vi "Configure List.vi"(0 "VISA resource name":refnum<visa-resource-name>, 1 "Amplitude Data":dbl[](array[numeric])=[1.0] format="%#.4g", 2 "Trigger Output Data":bool[](array[boolean]), 5 "List Type (0: Current)":u16(ring) items=["Current", "Dwell", "Frequency", "Frequency Slew Rate", "Phase", "Waveform", "Trigger Output", "Voltage", "Voltage Slew Rate", "Voltage Offset", "Voltage Offset Slew Rate"], 7 "List Repeat Count (1)":dbl=1.0, 9 "List Sequencing (0: Auto)":u16(ring) items=["Auto", "Once"], 11 "error in (no error)":errorcluster, 12 "Waveform Data":T1(array[cluster]) {"Shape (0: Sinusoid)" items=["Sinusoid", "Square", "Clipped Sinusoid", "User-Specified"]}) -> (4 "VISA resource name out":refnum<visa-resource-name>, 15 "error out":errorcluster)   [LabVIEW 2019, in "Agilent 681x Series.lvlib"]
doc: "Configures the lists of various parameters such as voltage, current or frequency for the instrument to use when list mode is selected for configuration of those parameters."
uses:
  <instrlib>/Agilent 681x Series/Agilent 681x Series.lvlib
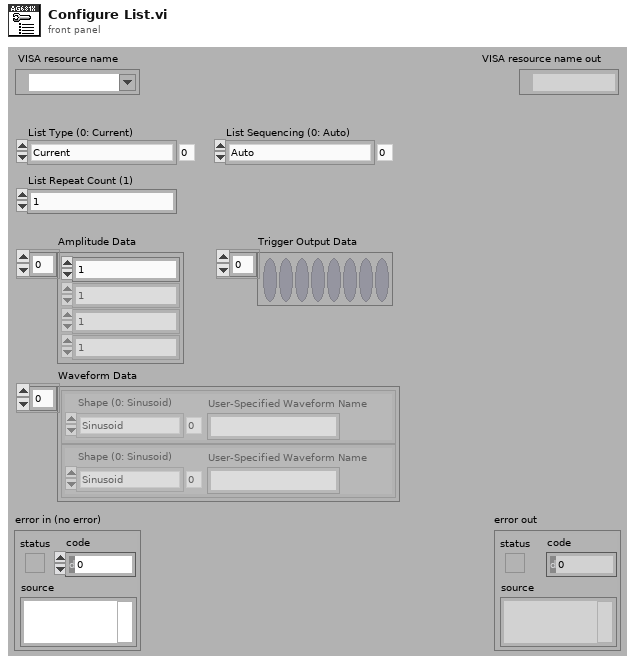
[diagram p1: front panel]
types:
  T1 = cluster{"Shape (0: Sinusoid)":u16, "User-Specified Waveform Name":string}[]
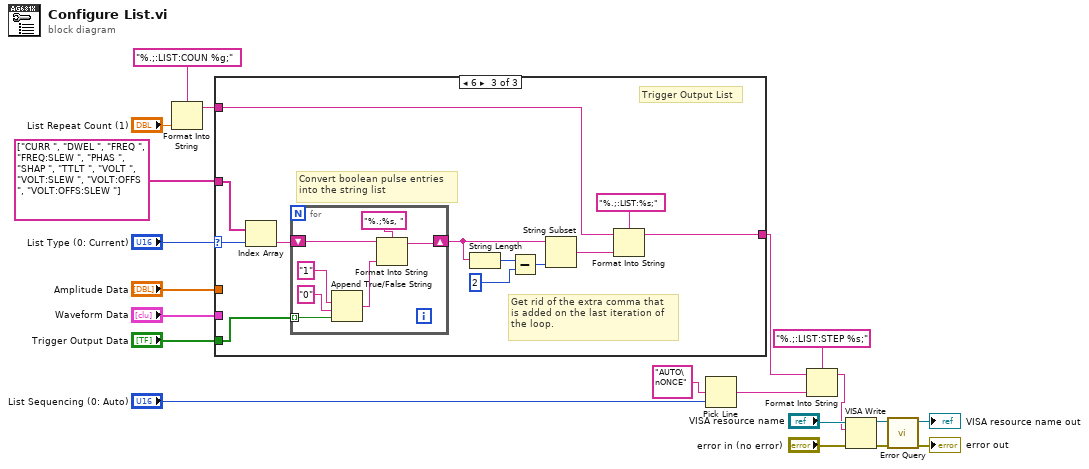
[diagram p0: block diagram]
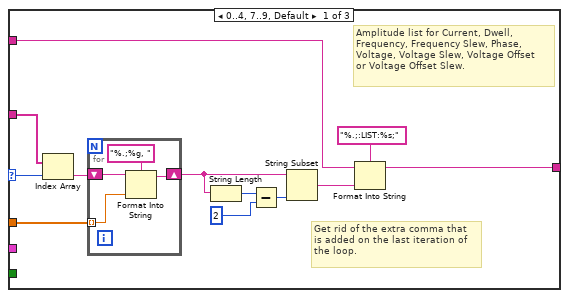
[diagram p2: hidden frame]
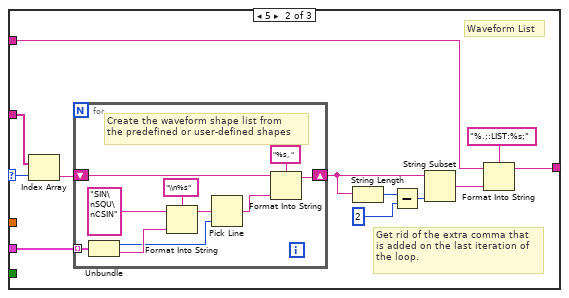
[diagram p3: hidden frame]
diagram:
  n1 = Format Into String(format string="%.;:LIST:COUN %g;", "List Repeat Count (1)") -> (resulting string=w8:string)  [unwired: 2 in, 1 out]
  n2 = case shown="6" "List Type (0: Current)" {
    selector: "List Type (0: Current)" -> [w32 w41 w62]
    tunnel: string[] ["CURR ", "DWEL ", "FREQ ", "FREQ:SLEW ", "PHAS ", "SHAP ", "TTLT ", "VOLT ", "VOLT:SLEW ", "VOLT:OFFS ", "VOLT:OFFS:SLEW "] -> [w31 w42 w61]
    tunnel: "Amplitude Data" -> [w23 _ _]
    tunnel: w8 -> [w22 w40 w60]
    tunnel: [w21 w38 w63] -> w7
    tunnel: "Trigger Output Data" -> [_ _ w59]
    tunnel: "Waveform Data" -> [_ w37 _]
    frame 0..4, 7..9, Default {
      # "Amplitude list for Current, Dwell,\nFrequency, Frequency Slew, Phase,\nVoltage, Voltage Slew, Voltage Offset \nor Voltage Offset Slew."
      # "Get rid of the extra comma that\nis added on the last iteration of\nthe loop."
      n3 = Index Array(array=w31, index=w32) -> (element=w24:string)
      n4 = for {
        tunnel: w23 -> [w35] mode=indexing
        shift-right: [w33] -> w25
        shift-left: w24 -> [w36]
        n5 = Format Into String(format string="%.;%g, ", initial string=w36, w35) -> (resulting string=w33:string)  [unwired: 1 in, 1 out]
      }
      n6 = String Length(string=w25) -> (length=w26:i32)
      n7 = Subtract(x=w26, y=2) -> (x-y=w28:i32)
      n8 = String Subset(string=w25, length (rest)=w28) -> (substring=w29:string)  [unwired: 1 in]
      n9 = Format Into String(format string="%.;:LIST:%s;", initial string=w22, w29) -> (resulting string=w21:string)  [unwired: 1 in, 1 out]
    }
    frame 5 {
      # "Waveform List"
      # "Get rid of the extra comma that\nis added on the last iteration of\nthe loop."
      n10 = Index Array(array=w42, index=w41) -> (element=w39:string)
      n11 = for {
        shift-right: [w56] -> w43
        shift-left: w39 -> [w58]
        tunnel: w37 -> [w55] mode=indexing
        # "Create the waveform shape list from\nthe predefined or user-defined shapes"
        n12 = Unbundle(w55) -> ("Shape (0: Sinusoid)"=w49:u16, "User-Specified Waveform Name"=w54:string)
        n13 = Format Into String(format string="\\n%s", initial string="SIN\nSQU\nCSIN", w54) -> (resulting string=w50:string)  [unwired: 1 in, 1 out]
        n14 = Pick Line(multi-line string=w50, line index=w49) -> (output string=w51:string)  [unwired: 1 in]
        n15 = Format Into String(format string="%s, ", initial string=w58, w51) -> (resulting string=w56:string)  [unwired: 1 in, 1 out]
      }
      n16 = String Length(string=w43) -> (length=w44:i32)
      n17 = Subtract(x=w44, y=2) -> (x-y=w46:i32)
      n18 = String Subset(string=w43, length (rest)=w46) -> (substring=w47:string)  [unwired: 1 in]
      n19 = Format Into String(format string="%.;:LIST:%s;", initial string=w40, w47) -> (resulting string=w38:string)  [unwired: 1 in, 1 out]
    }
    frame 6 {
      # "Get rid of the extra comma that\nis added on the last iteration of\nthe loop."
      # "Convert boolean pulse entries\ninto the string list"
      # "Trigger Output List"
      n20 = Index Array(array=w61, index=w62) -> (element=w64:string)
      n21 = for {
        shift-right: [w75] -> w65
        shift-left: w64 -> [w77]
        tunnel: w59 -> [w73] mode=indexing
        n22 = Append True/False String(1:w73, 2:"0" ("false string"), 3:"1" ("true string")) -> (0:w74:string)  [unwired: 1 in]
        n23 = Format Into String(format string="%.;%s, ", initial string=w77, w74) -> (resulting string=w75:string)  [unwired: 1 in, 1 out]
      }
      n24 = String Length(string=w65) -> (length=w66:i32)
      n25 = Subtract(x=w66, y=2) -> (x-y=w68:i32)
      n26 = String Subset(string=w65, length (rest)=w68) -> (substring=w69:string)  [unwired: 1 in]
      n27 = Format Into String(format string="%.;:LIST:%s;", initial string=w60, w69) -> (resulting string=w63:string)  [unwired: 1 in, 1 out]
    }
  }
  n28 = Pick Line(multi-line string="AUTO\nONCE", line index="List Sequencing (0: Auto)") -> (output string=w5:string)  [unwired: 1 in]
  n29 = Format Into String(format string="%.;:LIST:STEP %s;", initial string=w7, w5) -> (resulting string=w2:string)  [unwired: 1 in, 1 out]
  n30 = VISA Write(VISA resource name="VISA resource name", write buffer=w2, error in (no error)="error in (no error)") -> (VISA resource name out=w18:refnum<visa-resource-name>, error out=w17:errorcluster)  [unwired: 1 out]
  n31 = call <instrlib>:"Error Query.vi"("error in (no error)"=w17, "VISA resource name"=w18) -> ("error out"=→"error out":errorcluster, "VISA resource name out"=→"VISA resource name out":refnum<visa-resource-name>)  [unwired: 6 in, 2 out]
